vi "Remove_FF_lone_spikes.vi"(3 "ADC Frequency Hz":dbl=1000.0 format="%.2f", 4 "Bkgnd variance":dbl format="%.6f", 5 "AIC index":i32, 6 "Time Trace":dbl[](graph)) -> (0 "No Removed":i32, 2 "Filtered Time Trace":dbl[](graph))   [LabVIEW 2012]
uses:
  Globals/Meas_global.vi
  <vilib>/Analysis/NI_AALBase.lvlib
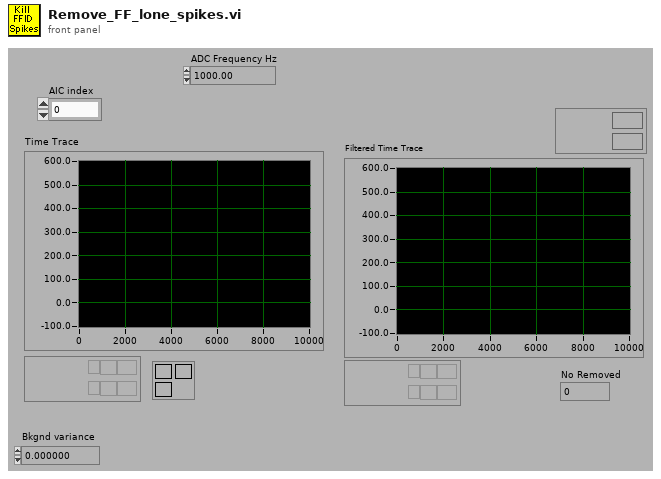
[diagram p1: front panel]
types:
  T1 = typedef "Analysis_info_cluster.ctl" = cluster{"Colour":u32, "Inst type":T2, "Inst name":string, "Symbol":string, "Code name":string, "Extra Info":string, "Inst Array":T3, "Extra Titles":string[], "Extra Values":string[], "U":dbl, "u^2":dbl, "u^3":dbl, "u^4":dbl, "Skew_u":dbl, "Kurt_u":dbl, "Sd Error in Mean":dbl, "% u'/U":dbl, "X":dbl, "Y":dbl, "Z":dbl, "Timescale integral to 25%":dbl, "Sd Error in Variance":dbl, "Calib File":path, "Calib Constants":dbl[], "Output Position":bool, "Full Stats":bool, "Av Sampling Rate":dbl, "Av No of Samples":dbl, "Total Meas Time (s)":dbl, "ADAM Ch Name":string}
  T2 = typedef "Inst_type.ctl" = enum16{"Propeller anemometer", "Raw voltage", "Pressure Transducer", "Pitot-static tube", "Preston tube", "Hot wire", "Cross wire 1", "Cross wire 2", "Generic Linear", "Generic Polynomial", "Generic BackPoly", "Fast FID", "Thermocouple", "Cold wire", "Pulsed Wire", "LDA Vel", "LDA Tran time", "LDA Arr time"}
  T3 = typedef "Instrument_Array.ctl" = enum16{"PWA", "LDA", "Analogue"}
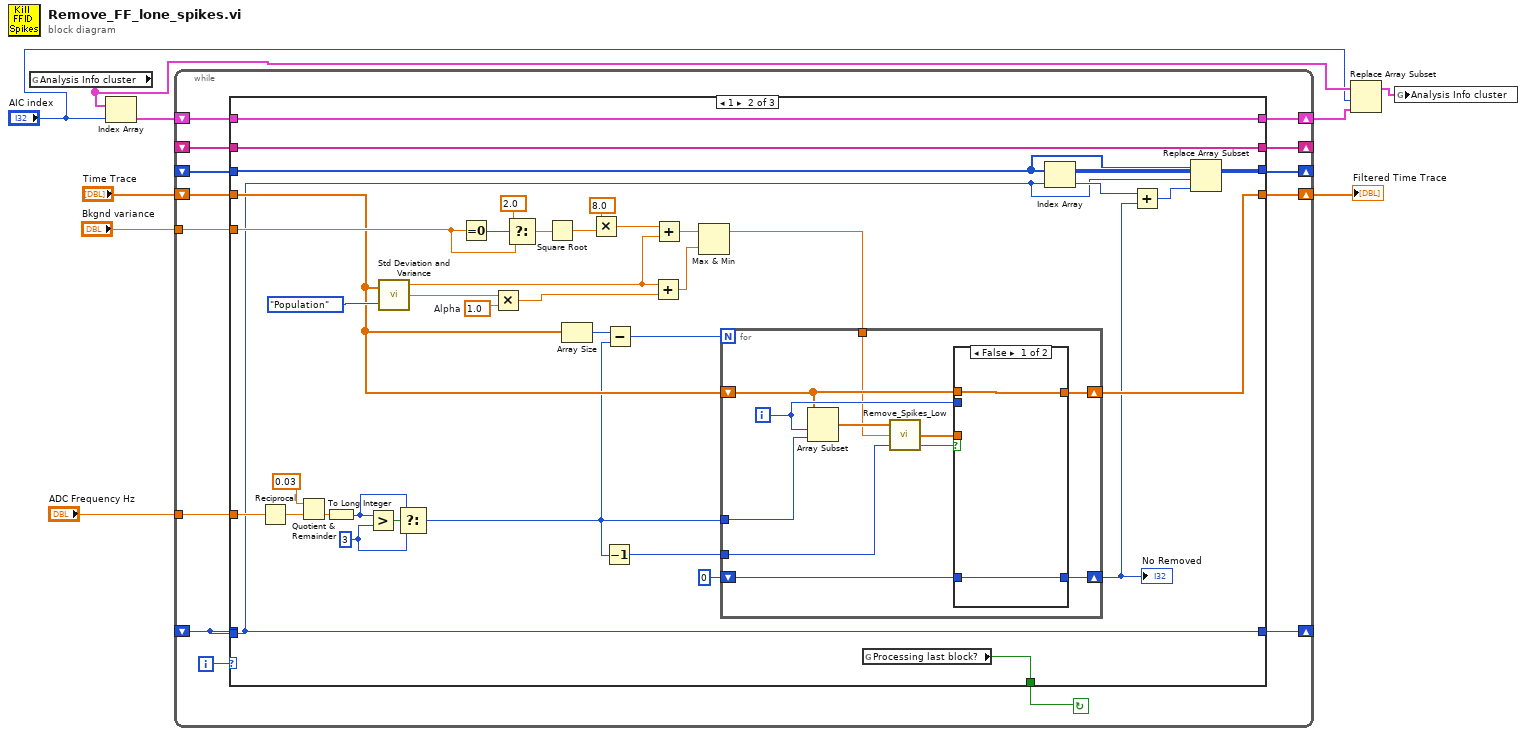
[diagram p0: block diagram]
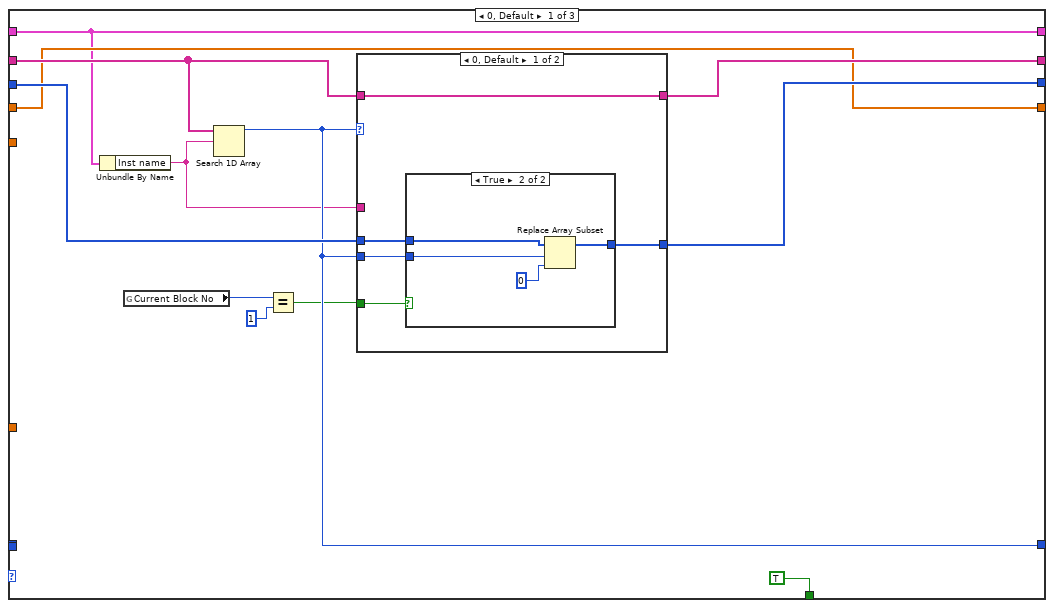
[diagram p2: hidden frame]
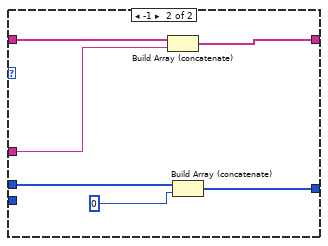
[diagram p4: hidden frame]
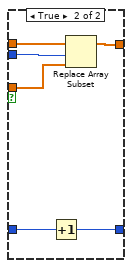
[diagram p5: hidden frame]
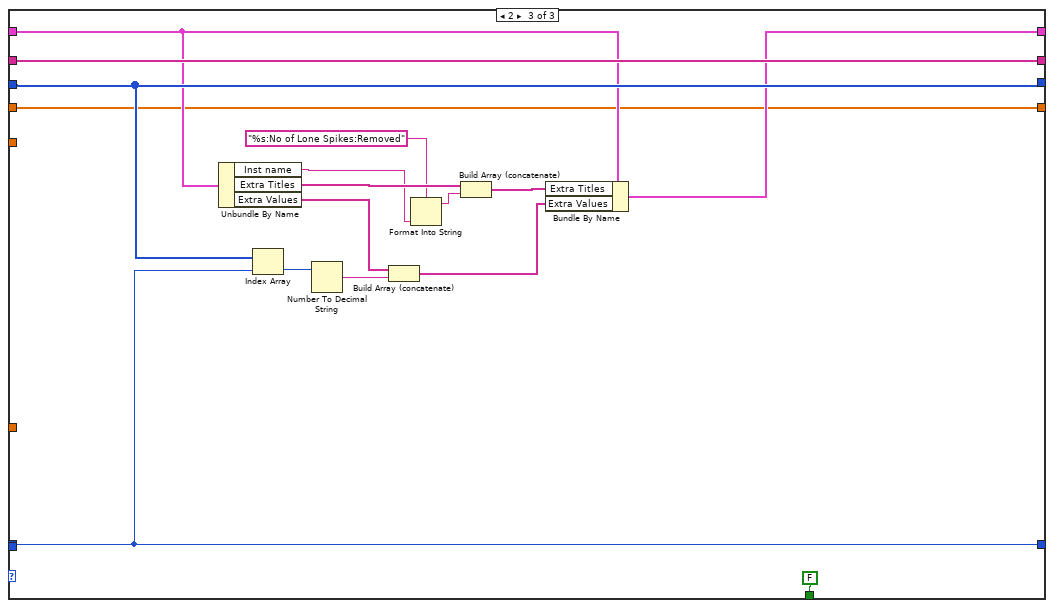
[diagram p6: hidden frame]
diagram:
  n1 = global read "Meas_global.vi" "Analysis Info cluster"() -> (w4:T1[])
  n2 = Index Array(array=w4, index="AIC index") -> (element=w5:T1)
  n3 = while {
    shift-left: _ -> [w20]
    shift-right: [w22] -> _
    shift-right: [w18] -> _
    shift-left: _ -> [w19]
    shift-right: [w16] -> _
    shift-left: _ -> [w17]
    shift-right: [w14] -> w3
    shift-left: w5 -> [w15]
    tunnel: "Bkgnd variance" -> [w13]
    shift-right: [w11] -> w7
    shift-left: "Time Trace" -> [w12]
    tunnel: "ADC Frequency Hz" -> [w10]
    i -> [w23]
    stop <- w21 continue-if-true
    n4 = case shown="1" w23 {
      tunnel: [w28 w66 w122] -> w22
      tunnel: [TRUE w64 FALSE ("Processing last block?")] -> w21
      tunnel: w20 -> [_ _ w122]
      tunnel: w20 -> [_ w66 _]
      tunnel: w19 -> [w32 w82 w120]
      tunnel: [w31 w82 w120] -> w18
      tunnel: w17 -> [w30 w81 w119]
      tunnel: [w29 w79 w119] -> w16
      tunnel: w15 -> [w25 w78 w116]
      tunnel: [w25 w78 w118] -> w14
      tunnel: w13 -> [_ w77 _]
      tunnel: w12 -> [w26 w70 w112]
      tunnel: [w26 w65 w112] -> w11
      tunnel: w10 -> [_ w75 _]
      frame 0, Default {
        n5 = Unbundle By Name(w25) -> ("Inst name"=w24:string)
        n6 = global read "Meas_global.vi" "Current Block No"() -> (w34:i32)
        n7 = Search 1D Array(1D array=w32, element=w24) -> (index of element=w28:i32)  [unwired: 1 out]
        n8 = Equal?(x=w34, y=1) -> (x = y?=w27:bool)
        n9 = case shown="0, Default" w28 {
          tunnel: w32 -> [w40 w51]
          tunnel: w24 -> [_ w50]
          tunnel: [w40 w49] -> w31
          tunnel: w30 -> [w39 w48]
          tunnel: [w38 w47] -> w29
          tunnel: w28 -> [w37 _]
          tunnel: w27 -> [w36 _]
          frame 0, Default {
            n10 = case shown="True" w36 {
              tunnel: w39 -> [w41 w45]
              tunnel: [w41 w44] -> w38
              tunnel: w37 -> [_ w43]
              frame False {
              }
              frame True {
                n11 = Replace Array Subset(array=w45, new element=0, index=w43) -> (w44:i32[])
              }
            }
          }
          frame -1 {
            n12 = Build Array (concatenate)(w51, w50) -> (w49:string[])
            n13 = Build Array (concatenate)(w48, 0) -> (w47:i32[])
          }
        }
      }
      frame 1 {
        w60 = 3 ("y")
        w54 = 1.0  # Alpha
        n14 = Reciprocal(x=w75) -> (1/x=w73:dbl)
        n15 = Quotient & Remainder(x=0.03, y=w73) -> (floor(x/y)=w72:dbl)  [unwired: 1 out]
        n16 = To Long Integer(number=w72) -> (32bit integer=w59:i32)
        n17 = Greater?(x=w59, y=w60) -> (0:w61:bool)
        n18 = call <vilib>:"Std Deviation and Variance.vi"("X"=w70, "Weighting (Sample)"=enum16{"Sample", "Population"}."Population") -> ("mean"=w56:dbl, "standard deviation"=w55:dbl)  [unwired: 1 out]
        n19 = Select(t=w59, s=w61, f=w60) -> (s? t:f=w58:i32)
        n20 = Equal To 0?(x=w77) -> (x = 0?=w88:bool)
        n21 = Multiply(x=w55, y=w54) -> (x*y=w57:dbl)
        n22 = Select(t=2.0, s=w88, f=w77) -> (s? t:f=w86:dbl)
        n23 = Square Root(x=w86) -> (sqrt(x)=w53:dbl)
        n24 = Array Size(array=w70) -> (size(s)=w69:i32)
        n25 = Multiply(x=8.0 ("y"), y=w53) -> (x*y=w89:dbl)
        n26 = Decrement(x=w58) -> (x-1=w71:i32)
        n27 = Subtract(x=w69, y=w58) -> (x-y=w68:i32)
        n28 = Add(x=w56, y=w57) -> (x+y=w83:dbl)
        n29 = Add(x=w89, y=w56) -> (x+y=w84:dbl)
        n30 = Max & Min(x=w84, y=w83) -> (max(x,y)=w67:dbl)  [unwired: 1 out]
        n31 = for {
          N: w68 -> [_]
          shift-right: [w93] -> w65
          shift-left: w70 -> [w94]
          tunnel: w58 -> [w100]
          tunnel: w71 -> [w99]
          tunnel: w67 -> [w92]
          shift-right: [w91] -> w63
          shift-left: 0 -> [w90]
          i -> [w96]
          n32 = Array Subset(array=w94, index=w96, length=w100) -> (w98:dbl[])
          n33 = call "Remove_Spikes_Low.vi"("index"=w99, "Background noise"=w92, "Time Trace"=w98) -> ("Spike"=w97:bool, "Filtered Time Trace"=w95:dbl[])  [unwired: 1 out]
          n34 = case shown="False" w97 {
            tunnel: w96 -> [_ w108]
            tunnel: w95 -> [_ w107]
            tunnel: w94 -> [w102 w106]
            tunnel: [w102 w105] -> w93
            tunnel: [w101 w103] -> w91
            tunnel: w90 -> [w101 w104]
            frame False {
            }
            frame True {
              n35 = Increment(x=w104) -> (x+1=w103:i32)
              n36 = Replace Array Subset(array=w106, new element=w107, index=w108) -> (w105:dbl[])
            }
          }
        }
        "No Removed" <- w63
        n37 = global read "Meas_global.vi" "Processing last block?"() -> (w64:bool)
        n38 = Index Array(array=w81, index=w66) -> (element=w80:i32)
        n39 = Add(x=w80, y=w63) -> (x+y=w76:i32)
        n40 = Replace Array Subset(array=w81, new element=w76, index=w66) -> (w79:i32[])
      }
      frame 2 {
        n41 = Unbundle By Name(w116) -> ("Inst name"=w110:string, "Extra Titles"=w115:string[], "Extra Values"=w114:string[])
        n42 = Index Array(array=w119, index=w122) -> (element=w121:i32)
        n43 = Number To Decimal String(number=w121) -> (decimal integer string=w123:string)  [unwired: 1 out]
        n44 = Build Array (concatenate)(w114, w123) -> (w113:string[])
        n45 = Format Into String(format string="%s:No of Lone Spikes:Removed", w110) -> (resulting string=w111:string)  [unwired: 2 in, 1 out]
        n46 = Build Array (concatenate)(w115, w111) -> (w117:string[])
        n47 = Bundle By Name(cluster=w116, "Extra Titles"=w117, "Extra Values"=w113) -> (w118:T1)
      }
    }
  }
  "Filtered Time Trace" <- w7
  n48 = Replace Array Subset(array=w4, new element=w3, index="AIC index") -> (w1:T1[])
  n49 = global write "Meas_global.vi" "Analysis Info cluster"(w1) -> ()
